vi "SaveZSpec.vi"() -> ()   [LabVIEW 2014]
uses:
  <userlib>/Nanonis Prog Interface V5/Nanonis Prog Interface.lvlib
panel:
  in  "milliseconds to wait":u32=500
  in  "Bias (V)":sgl=-0.00027 format="%#_5p"
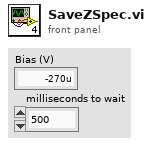
[diagram p1: front panel]
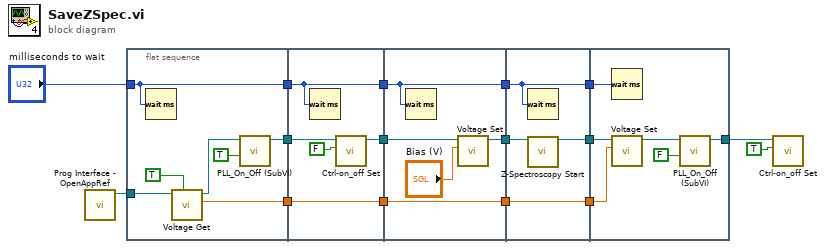
[diagram p0: block diagram]
diagram:
  n1 = call <userlib>:"Prog Interface - OpenAppRef.vi"() -> ("Application reference"=w16:refnum<vi>)  [unwired: 6 in, 1 out]
  n2 = flat-sequence {
    tunnel: w16 -> [w21]
    tunnel: "milliseconds to wait" -> [w18]
    tunnel: [w20] -> w9
    tunnel: [w19] -> w8
    tunnel: [w18] -> w6
    tunnel: w9 -> [w25]
    tunnel: w8 -> [w28]
    tunnel: [w28] -> w7
    tunnel: w6 -> [w27]
    tunnel: [w27] -> w5
    tunnel: [w26] -> w4
    tunnel: [w31] -> w14
    tunnel: w7 -> [w30]
    tunnel: [w30] -> w12
    tunnel: w5 -> [w29]
    tunnel: [w29] -> w10
    tunnel: w4 -> [w32]
    tunnel: w14 -> [w37]
    tunnel: [w36] -> w13
    tunnel: w12 -> [w35]
    tunnel: [w35] -> w11
    tunnel: w10 -> [w34]
    tunnel: [w34] -> w3
    tunnel: w13 -> [w43]
    tunnel: w11 -> [w42]
    tunnel: w3 -> [w39]
    tunnel: [w38] -> w2
    frame #0 {
      n3 = Wait (ms)(milliseconds to wait=w18) -> ()  [unwired: 1 out]
      n4 = call <userlib>:"Voltage Get.vi"("Wait for newest data (F)"=TRUE, "Application ref in"=w21) -> ("Bias (V)"=w19:sgl, "Application ref out"=w23:refnum<vi>)  [unwired: 7 in, 1 out]
      n5 = call "PLL_On_Off (SubVI).vi"("Output ON/OFF (F=OFF)"=TRUE, "Application in"=w23) -> ("Application out"=w20:refnum<vi>)  [unwired: 8 in, 1 out]
    }
    frame #1 {
      n6 = Wait (ms)(milliseconds to wait=w27) -> ()  [unwired: 1 out]
      n7 = call <userlib>:"Ctrl-on_off Set.vi"("Z Controller ON/OFF"=FALSE, "Application ref in"=w25) -> ("Application ref out"=w26:refnum<vi>)  [unwired: 8 in, 1 out]
    }
    frame #2 {
      n8 = Wait (ms)(milliseconds to wait=w29) -> ()  [unwired: 1 out]
      n9 = call <userlib>:"Voltage Set.vi"("Bias (V)"="Bias (V)", "Application ref in"=w32) -> ("Application ref out"=w31:refnum<vi>)  [unwired: 8 in, 1 out]
    }
    frame #3 {
      n10 = Wait (ms)(milliseconds to wait=w34) -> ()  [unwired: 1 out]
      n11 = call <userlib>:"Z-Spectroscopy Start.vi"("Application ref in"=w37) -> ("Application ref out"=w36:refnum<vi>)  [unwired: 10 in, 4 out]
    }
    frame #4 {
      n12 = Wait (ms)(milliseconds to wait=w39) -> ()  [unwired: 1 out]
      n13 = call <userlib>:"Voltage Set.vi"("Bias (V)"=w42, "Application ref in"=w43) -> ("Application ref out"=w41:refnum<vi>)  [unwired: 8 in, 1 out]
      n14 = call "PLL_On_Off (SubVI).vi"("Output ON/OFF (F=OFF)"=FALSE, "Application in"=w41) -> ("Application out"=w38:refnum<vi>)  [unwired: 8 in, 1 out]
    }
  }
  n15 = call <userlib>:"Ctrl-on_off Set.vi"("Z Controller ON/OFF"=TRUE, "Application ref in"=w2) -> ()  [unwired: 8 in, 2 out]
